vi "Write.vi"(6 "Close (F)":bool, 9 "timeout in ms (-1)":i32=-1, 10 "Element":T1, 11 "Writer in":refnum<class "Writer.lvclass">) -> (1 "timed out?":bool, 4 "Closed?":bool)   [LabVIEW 2022 SP3, in "Enclave.lvlib" / "Writer.lvclass"]
uses:
  Writer.lvclass
  Element.ctl
  Writer.lvclass/Writer.ctl
  Enclave/Enclave.lvclass/Enclave.ctl
  Enclave/Check Ready.vi
  Enclave/Enclave.lvclass
  Enclave.lvlib
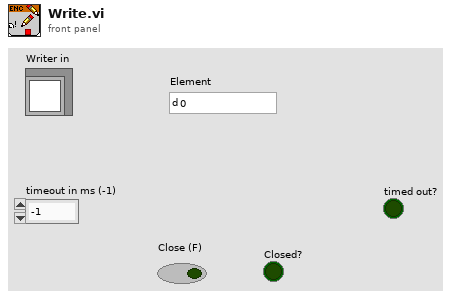
[diagram p1: front panel]
types:
  T1 = typedef "Enclave.lvlib/Element.ctl" = dbl
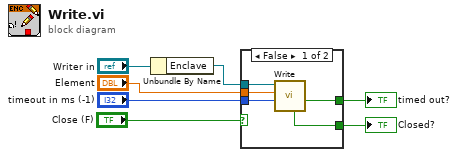
[diagram p0: block diagram]
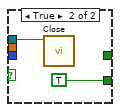
[diagram p2: hidden frame]
diagram:
  n1 = Unbundle By Name("Writer in") -> ("Enclave"=w6:refnum<class "Enclave.lvclass">)
  n2 = case shown="False" "Close (F)" {
    tunnel: w6 -> [w12 w14]
    tunnel: "Element" -> [w11 _]
    tunnel: "timeout in ms (-1)" -> [w10 _]
    tunnel: [w9 _] -> w3
    tunnel: [w8 TRUE ("Closed?")] -> w1
    frame False {
      n3 = call "Write.vi"("timeout in ms (-1)"=w10, "Element"=w11, "Enclave in"=w12) -> ("timed out?"=w9:bool, "Closed?"=w8:bool)  [unwired: 7 in]
    }
    frame True {
      n4 = call "Close.vi"("Enclave in"=w14) -> ()  [unwired: 11 in]
    }
  }
  "timed out?" <- w3
  "Closed?" <- w1
